vi "sendStop.vi"(8 "error in (no error)":errorcluster, 10 "stop":enum16{"stopBeforeNext", "stopNow"}(ring), 11 "ExperimentControlEvents in":refnum<class "ExperimentControlEvents.lvclass">) -> (0 "error out":errorcluster, 3 "ExperimentControlEvents out":refnum<class "ExperimentControlEvents.lvclass">)   [LabVIEW 2011, in "Views.lvlib" / "ExperimentControl.lvlib" / "ExperimentControlEvents.lvclass"]
uses:
  ExperimentControlEvents.lvclass
  ExperimentControlEvents.lvclass/ExperimentControlEvents.ctl
  Events/Event.lvclass
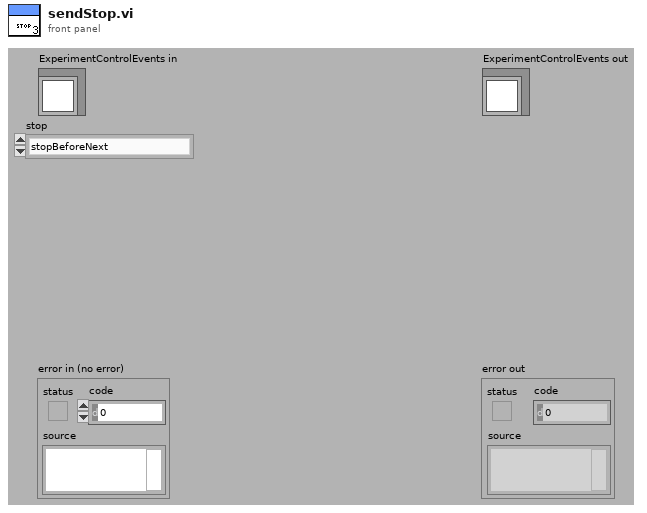
[diagram p1: front panel]
types:
  T1 = enum16{"close", "stopRunning", "runSingleScript", "runExperiment", "runExperimentScript"}
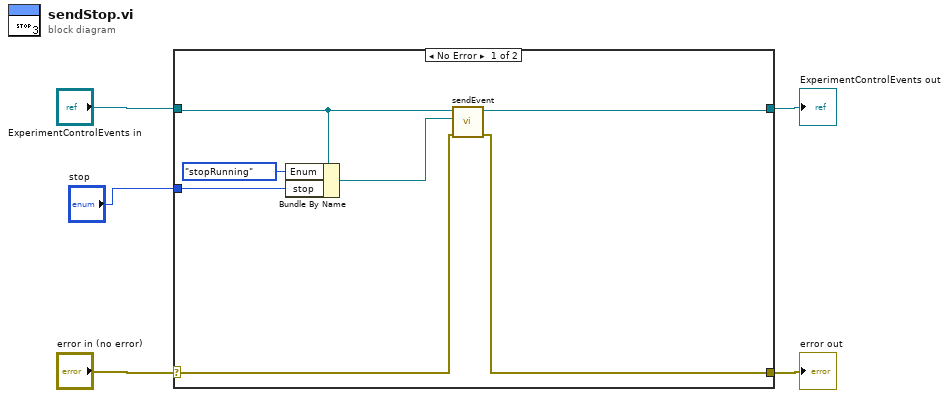
[diagram p0: block diagram]
diagram:
  n1 = case shown="No Error" "error in (no error)" {
    selector: "error in (no error)" -> [w8 w14]
    tunnel: [w7 w14] -> w2
    tunnel: [w12 w13] -> w5
    tunnel: "ExperimentControlEvents in" -> [w11 w13]
    tunnel: "stop" -> [w6 _]
    frame No Error {
      n2 = Bundle By Name(cluster=w11, "Enum"=T1."stopRunning", "stop"=w6) -> (w10:refnum<class "ExperimentControlEvents.lvclass">)
      n3 = call "sendEvent.vi"("error in (no error)"=w8, "data"=w10, "Event in"=w11) -> ("error out"=w7:errorcluster, "Event out"=w12:refnum<class "ExperimentControlEvents.lvclass">)  [unwired: 7 in]
    }
    frame Error {
    }
  }
  "error out" <- w2
  "ExperimentControlEvents out" <- w5
